vi "Add Section Node.vi"(9 "Type Name":string, 10 "Code Documentation":string, 11 "Doc Ref":refnum<k20>) -> (2 "Updated Node Ref":refnum<k20>)   [LabVIEW 2025]
uses:
  Types/New Node Types.ctl
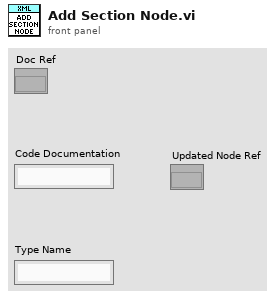
[diagram p1: front panel]
types:
  T1 = typedef "New Node Types.ctl" = enum16{"Channel", "Waveform", "Section"}
  T2 = cluster{"Tag Name":string, "Code Documentation":string}
  T3 = cluster{"Tag Name":string, "Code Documentation":string}[]
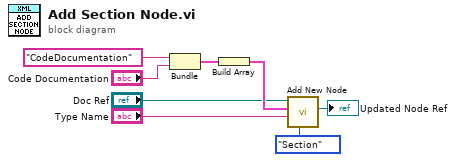
[diagram p0: block diagram]
diagram:
  n1 = Bundle("Tag Name"="CodeDocumentation", "Code Documentation"="Code Documentation") -> (w6:T2)  [unwired: 1 in]
  n2 = Build Array(w6) -> (w5:T3)
  n3 = call "Add New Node.vi"("New Node Types"=New_Node_Types."Section", "Type Name"="Type Name", "Text Nodes"=w5, "Doc Ref"="Doc Ref") -> ("Updated Node Ref"=→"Updated Node Ref":refnum<k20>)  [unwired: 7 in]
